vi "Key Pressed.vi"(8 "error in (no error)":errorcluster, 10 "Key Pressed":i32, 11 "Numeric in":refnum<class "Numeric.lvclass">) -> (0 "error out":errorcluster, 3 "Numeric out":refnum<class "Numeric.lvclass">)   [LabVIEW 2020, in "Keypad.lvlib" / "Numeric.lvclass"]
uses:
  Numeric.lvclass
  Keypad/Keypad.lvclass
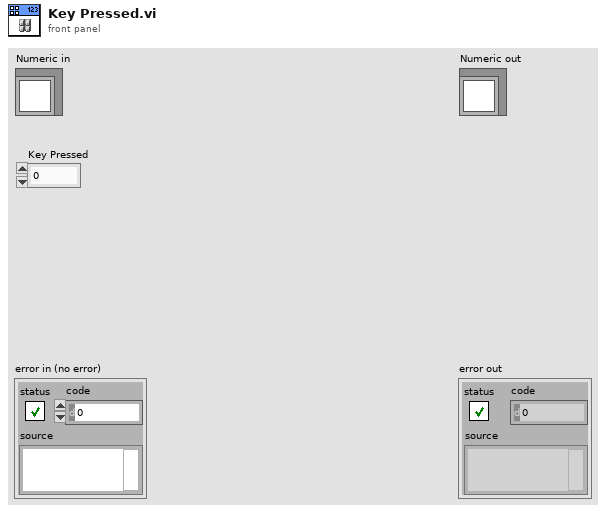
[diagram p1: front panel]
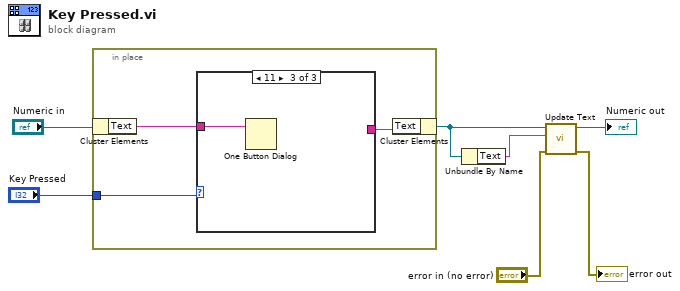
[diagram p0: block diagram]
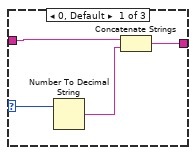
[diagram p2: hidden frame]
diagram:
  n1 = in-place {
    in-place-border: "Key Pressed" -> [w9]
    n2 = in-place-cluster #1("Numeric in") -> ("Text"=w10:string)
    n3 = case shown="11" w9 {
      selector: w9 -> [w14 _ _]
      tunnel: w10 -> [w13 _ w15]
      tunnel: [w11 _ _] -> w8
      frame 0, Default {
        n4 = Number To Decimal String(number=w14) -> (decimal integer string=w12:string)  [unwired: 1 in]
        n5 = Concatenate Strings(w13, w12) -> (w11:string)
      }
      frame 10 {
        # "Clears the text display"
      }
      frame 11 {
        n6 = One Button Dialog(message=w15) -> ()  [unwired: 1 in, 1 out]
      }
    }
    n7 = in-place-cluster #1("Text"=w8) -> (w4:refnum<class "Numeric.lvclass">)
  }
  n8 = Unbundle By Name(w4) -> ("Text"=w5:string)
  n9 = call "Update Text.vi"("error in (no error)"="error in (no error)", "Text"=w5, "Keypad in"=w4) -> ("error out"=→"error out":errorcluster, "Keypad out"=→"Numeric out":refnum<class "Numeric.lvclass">)  [unwired: 7 in]
